vi "Zero Origin.vi"(8 "error in":errorcluster, 11 "Flex UI in":refnum<class "Flex UI.lvclass">) -> (0 "error out":errorcluster, 3 "Flex UI out":refnum<class "Flex UI.lvclass">)   [LabVIEW 2016, in "Flex UI.lvclass"]
uses:
  Flex UI.lvclass
  <vilib>/Utility/miscctls.llb/LVPointTypeDef.ctl
  Flex UI.lvclass/Flex UI.ctl
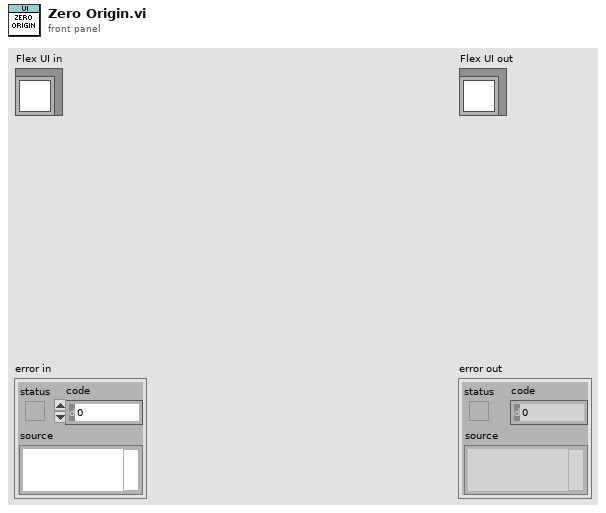
[diagram p1: front panel]
types:
  T1 = typedef "LVPointTypeDef.ctl" = cluster{"Horizontal":i16, "Vertical":i16}
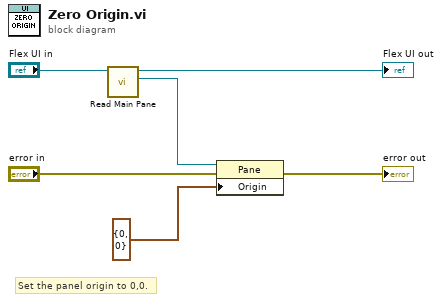
[diagram p0: block diagram]
diagram:
  # "Set the panel origin to 0,0."
  n1 = call "Read Main Pane.vi"("Flex UI in"="Flex UI in") -> ("Main Pane"=w1:refnum<vi>, "Flex UI out"=→"Flex UI out":refnum<class "Flex UI.lvclass">)  [unwired: 9 in]
  n2 = property class="Pane"(reference=w1, error in="error in", "Origin"=T1 {"Horizontal"=0, "Vertical"=0}) -> (error out=→"error out":errorcluster)  [unwired: 1 out]
